vi "IF Reading.vi"(8 "error constant":errorcluster) -> (0 "error constant 2":errorcluster, 3 "IF readings (meters)":dbl[](array[numeric]) format="%_6g")   [LabVIEW 2016]
uses:
  <vilib>/myRIO/Express VI/Onboard IO/AI/AI Express VI.xnode
  <vilib>/myRIO/Instrument Drivers/Onboard IO/AI/vis/Read.vi
  <vilib>/myRIO/Instrument Drivers/Onboard IO/AI/AI.lvlib
  <vilib>/myRIO/Common/Instrument Driver Framework/Utilities/typedefs/Analog Scaling Constants.ctl
  <vilib>/myRIO/Common/Instrument Driver Framework/Utilities/typedefs/Analog Scaling Constants List.ctl
  <vilib>/myRIO/Common/Instrument Driver Framework/myRIO v1.0/AI/typedefs/AI Channels Enum.ctl
  <vilib>/myRIO/Common/Instrument Driver Framework/myRIO v1.0/AI/typedefs/AI Channels List.ctl
  <vilib>/myRIO/Common/Instrument Driver Framework/Utilities/typedefs/Generic FPGA Reference.ctl
  <vilib>/myRIO/Common/Instrument Driver Framework/Utilities/typedefs/myRIO v1.0 Reference.ctl
  <vilib>/myRIO/Common/Instrument Driver Framework/Utilities/typedefs/Hardware Version Enum.ctl
  <vilib>/myRIO/Common/Instrument Driver Framework/Utilities/typedefs/myRIO Generic Hardware Reference.ctl
  <vilib>/myRIO/Instrument Drivers/Onboard IO/AI/typedefs/AI Reference.ctl
  <vilib>/myRIO/Instrument Drivers/Onboard IO/AI/vis/myRIO AI Open.xnode
  <vilib>/myRIO/Common/Instrument Driver Framework/Utilities/vis/Is FPGA Ref Available.vi
  <vilib>/gmath/NI_Gmath.lvlib
  <vilib>/myRIO/Common/Instrument Driver Framework/myRIO v1.0/AI/vis/myRIO v1.1 Open AI.vi
  <vilib>/userdefined/High Color/nirio_resource_hc.ctl
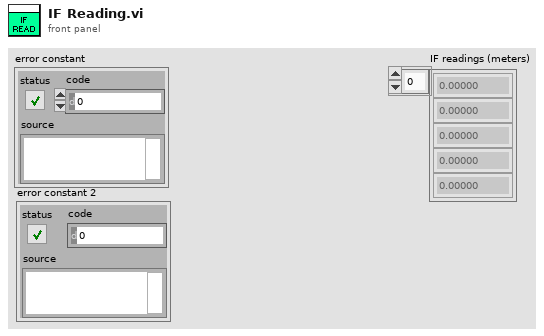
[diagram p1: front panel]
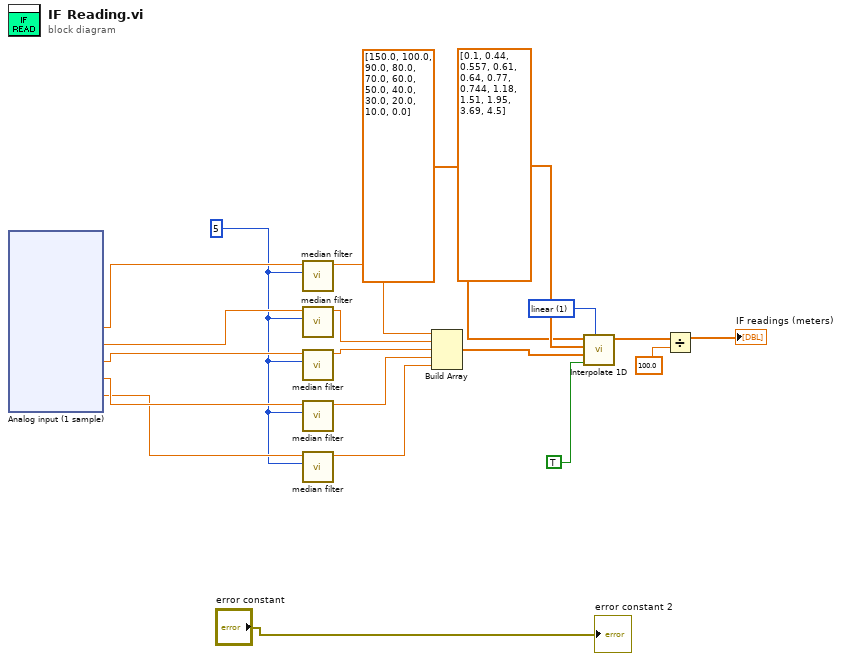
[diagram p0: block diagram]
diagram:
  w4 = 1 items=["nearest", "linear", "spline", "cubic Hermite", "Lagrange"] ("method")
  w15 = 5 ("Sample Length")
  n1 = xnode "Analog input (1 sample)"() -> ("A/AI0 (Pin 3)"=w20:dbl, "A/AI1 (Pin 5)"=w19:dbl, "A/AI2 (Pin 7)"=w18:dbl, "A/AI3 (Pin 9)"=w17:dbl, "B/AI0 (Pin 3)"=w16:dbl)  [unwired: 1 in, 1 out]
  n2 = call "median filter.vi"("Sample Length"=w15, "Element Input"=w20) -> ("Output Element"=w14:dbl)  [unwired: 9 in]
  n3 = call "median filter.vi"("Sample Length"=w15, "Element Input"=w19) -> ("Output Element"=w13:dbl)  [unwired: 9 in]
  n4 = call "median filter.vi"("Sample Length"=w15, "Element Input"=w18) -> ("Output Element"=w12:dbl)  [unwired: 9 in]
  n5 = call "median filter.vi"("Sample Length"=w15, "Element Input"=w17) -> ("Output Element"=w11:dbl)  [unwired: 9 in]
  n6 = call "median filter.vi"("Sample Length"=w15, "Element Input"=w16) -> ("Output Element"=w10:dbl)  [unwired: 9 in]
  n7 = Build Array(w14, w13, w12, w11, w10) -> (w8:dbl[])
  n8 = call <vilib>:"Interpolate 1D.vi"("method"=w4, "X is monotonic"=TRUE, "xi"=w8, "X"=dbl[] [0.1, 0.44, 0.557, 0.61, 0.64, 0.77, 0.744, 1.18, 1.51, 1.95, 3.69, 4.5] ("Y"), "Y"=dbl[] [150.0, 100.0, 90.0, 80.0, 70.0, 60.0, 50.0, 40.0, 30.0, 20.0, 10.0, 0.0] ("X")) -> ("yi"=w5:dbl[])  [unwired: 4 in, 2 out]
  n9 = Divide(x=w5, y=100.0) -> (x/y=→"IF readings (meters)":dbl[])
  "error constant 2" <- "error constant"
